vi "Read data.vi"(8 "error in (no error)":errorcluster, 10 "Buffer mode":T1, 11 "ScopeBase In":refnum<class "ScopeBase.lvclass">) -> (0 "error out":errorcluster, 1 "Any read?":bool, 2 "Data":dbl[][](array[numeric]), 3 "ScopeBase Out":refnum<class "ScopeBase.lvclass">, 4 "FFT buffer":dbl[][](array[numeric]))   [LabVIEW 2018, in "ScopeBase.lvclass"]
uses:
  ScopeBase.lvclass
  controls/Data_display_mode.ctl
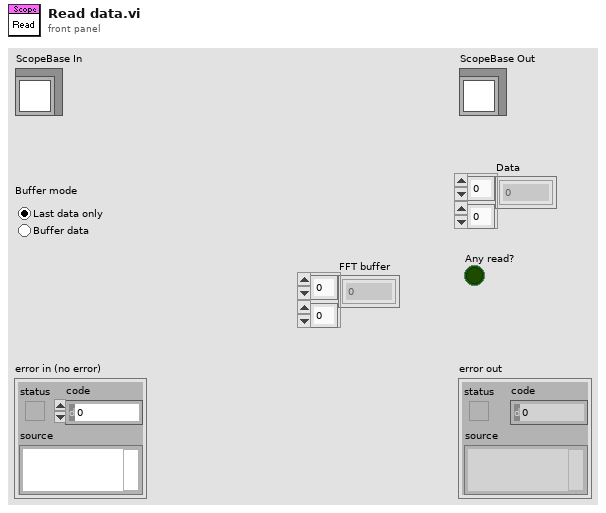
[diagram p1: front panel]
types:
  T1 = typedef "Data_display_mode.ctl" = enum32{"Last data only", "Buffer data"}
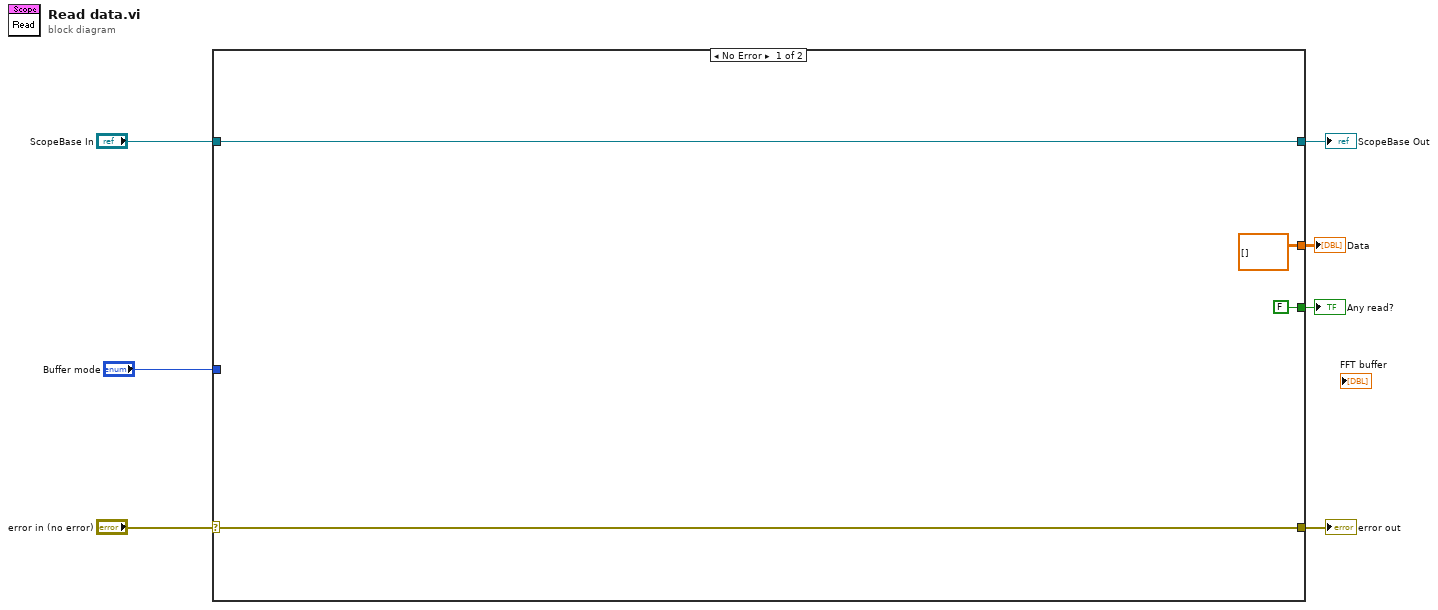
[diagram p0: block diagram]
diagram:
  n1 = case shown="No Error" "error in (no error)" {
    selector: "error in (no error)" -> [w11 w13]
    tunnel: [w11 w13] -> w6
    tunnel: [w10 w12] -> w4
    tunnel: "ScopeBase In" -> [w10 w12]
    tunnel: "Buffer mode" -> [_ _]
    tunnel: [dbl[][] [] ("Data") _] -> w1
    tunnel: [FALSE _] -> w2
    frame No Error {
    }
    frame Error {
    }
  }
  "error out" <- w6
  "ScopeBase Out" <- w4
  "Any read?" <- w2
  "Data" <- w1
